vi "YYYYMMDDHHMMSS.vi"(11 "seconds since 1Jan1904":timestamp) -> (3 "result string":string)   [LabVIEW 2019]
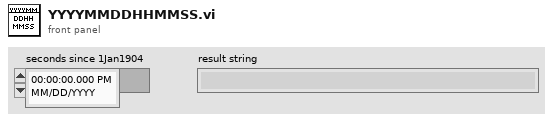
[diagram p1: front panel]
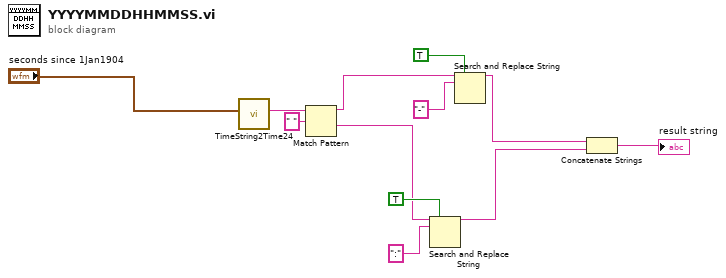
[diagram p0: block diagram]
diagram:
  n1 = call "TimeString2Time24.vi"("Time Stamp"="seconds since 1Jan1904") -> ("時間字串"=w1:string)  [unwired: 9 in, 1 out]
  n2 = Match Pattern(string=w1, regular expression=" ") -> (before substring=w6:string, after substring=w10:string)  [unwired: 1 in, 2 out]
  n3 = Search and Replace String(replace all?=TRUE ("replace all? (F)"), input string=w10, search string=":") -> (result string=w4:string)  [unwired: 5 in, 3 out]
  n4 = Search and Replace String(replace all?=TRUE ("replace all? (F)"), input string=w6, search string="-") -> (result string=w5:string)  [unwired: 5 in, 3 out]
  n5 = Concatenate Strings(w5, w4) -> (→"result string":string)
